vi "setControlTargetPosition.vi"(8 "error":errorcluster, 9 "target":dbl format="%#_13g", 10 "axis":i32, 11 "connection ID":refnum<k5>) -> (0 "error out":errorcluster, 2 "axis_out":i32, 3 "connection ID out":refnum<k5>)   [LabVIEW 2016, in "amc_api.lvlib"]
doc: "This function sets the target position for the movement on the selected axis."
uses:
  amc_api.lvlib
panel:
  out "jsonRespIn":string
  out "JSON-response":string="{\"jsonrpc\":\"2.0\",\"method\":\"\",\"params\":[5,1.245,true,\"name\"],\"id\":\"1\"}"
  out "JSON request":string
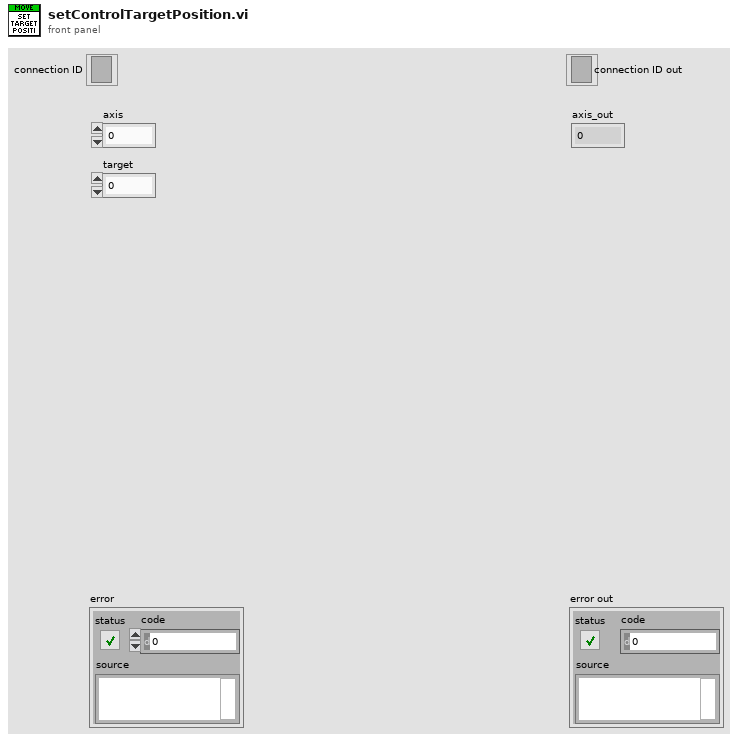
[diagram p1: front panel]
types:
  T1 = cluster{"jsonrpc":string, "method":string, "params":string[], "id":string, "api":i32, "pid":string}
  T2 = enum16{"Standard", "Buffered", "CRLF", "Immediate"}
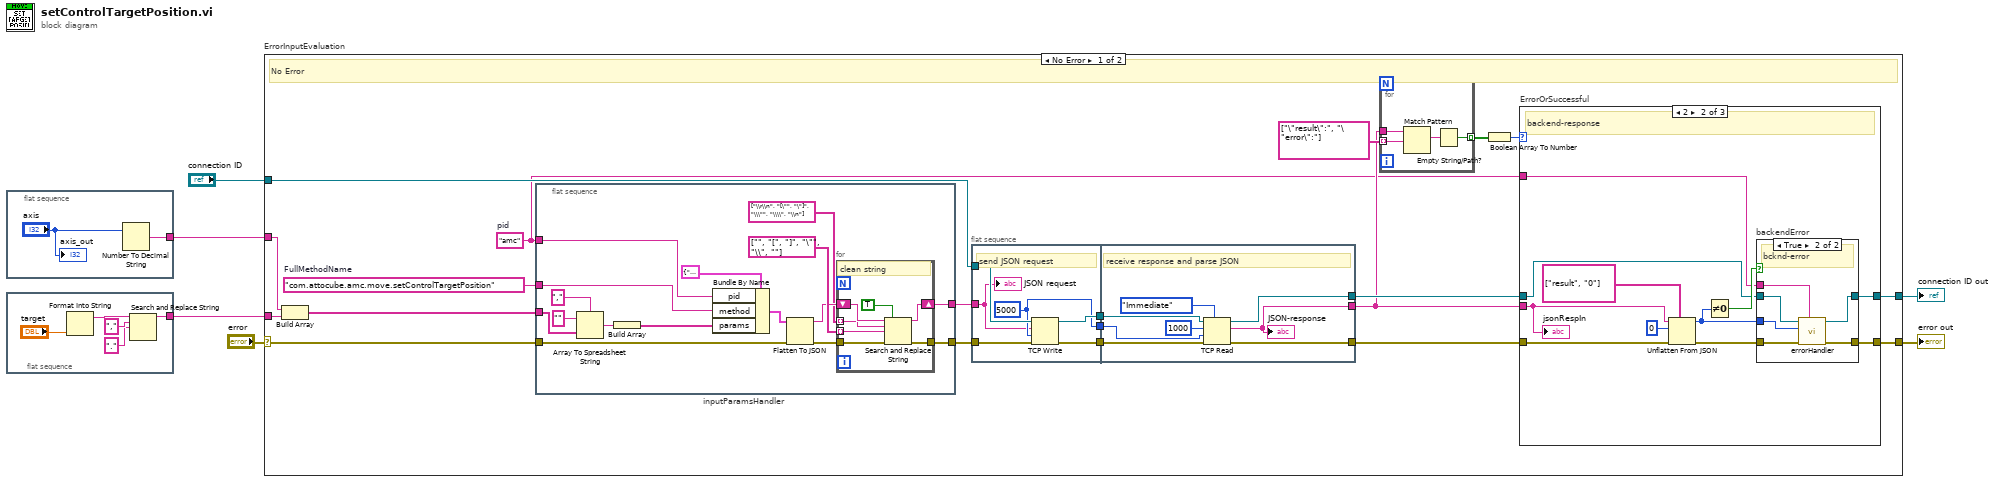
[diagram p0: block diagram]
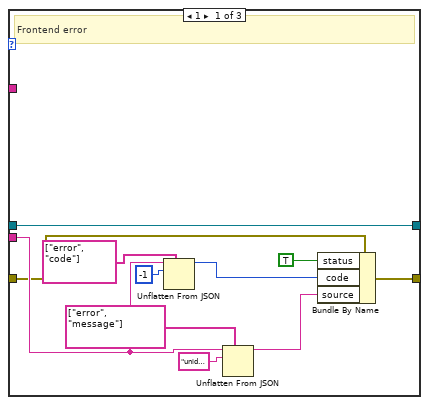
[diagram p2: hidden frame]
diagram:
  n1 = flat-sequence "in_axis" {
    tunnel: [w8] -> w2
    frame #0 {
      n2 = Number To Decimal String(number="axis") -> (decimal integer string=w8:string)  [unwired: 1 in]
      "axis_out" <- "axis"
    }
  }
  n3 = flat-sequence "in_double" {
    tunnel: [w9] -> w1
    frame #0 {
      n4 = Format Into String("target") -> (resulting string=w12:string)  [unwired: 3 in, 1 out]
      n5 = Search and Replace String(input string=w12, search string=",", replace string="." ("search string")) -> (result string=w9:string)  [unwired: 5 in, 3 out]
    }
  }
  n6 = case "ErrorInputEvaluation" shown="No Error" "error" {
    selector: "error" -> [w20 w107]
    tunnel: "connection ID" -> [w30 w108]
    tunnel: [w22 w107] -> w5
    tunnel: [w23 w108] -> w4
    tunnel: w2 -> [w15 _]
    tunnel: w1 -> [w14 _]
    frame No Error {
      w16 = "amc"  # pid
      w21 = "com.attocube.amc.move.setControlTargetPosition"  # FullMethodName
      # "No Error"
      n7 = Build Array ("ParametersArrayString")(w15, w14) -> (w19:string[])
      n8 = flat-sequence "inputParamsHandler" {
        tunnel: [w39] -> w18
        tunnel: w19 -> [w45]
        tunnel: w20 -> [w44]
        tunnel: [w41] -> w17
        tunnel: w21 -> [w35]
        tunnel: w16 -> [w34]
        frame #0 {
          n9 = Array To Spreadsheet String(delimiter (Tab)=",", array=w45, 3:"" ("format string")) -> (spreadsheet string=w47:string)
          n10 = Build Array "Build Array"(w47) -> (w36:string[])
          n11 = Bundle By Name(cluster=T1 {"jsonrpc"="2.0", "method"="com.attocube.amc.res.setRESReadOutFreq", "params"=[], "id"="1", "api"=2, "pid"=""}, "pid"=w34, "method"=w35, "params"=w36) -> (w46:T1)
          n12 = Flatten To JSON(anything=w46, error in (no error)=w44) -> (JSON string=w40:string, 11:w42:errorcluster)  [unwired: 1 in]
          n13 = for {
            tunnel: string[] ["\\r\\n", "[\"", "\"]", "\\\"", "\\\\", "\\n"] ("search string") -> [w53] mode=indexing
            tunnel: string[] ["", "[", "]", "\"", "\\", ""] ("replace string (\"\")") -> [w52] mode=indexing
            shift-right: [w55] -> w39
            shift-left: w40 -> [w54]
            tunnel: w42 -> [w51]
            tunnel: [w50] -> w41
            # "clean string"
            n14 = Search and Replace String(replace all?=TRUE ("replace all? (F)"), input string=w54, search string=w53, replace string=w52, error in=w51) -> (result string=w55:string, error out=w50:errorcluster)  [unwired: 3 in, 2 out]
          }
        }
      }
      n15 = flat-sequence {
        tunnel: w30 -> [w98]
        tunnel: [w96] -> w33
        tunnel: [w97] -> w32
        tunnel: w17 -> [w93]
        tunnel: [w95] -> w31
        tunnel: w18 -> [w94]
        tunnel: [w102] -> w26
        tunnel: w33 -> [w104]
        tunnel: w32 -> [w103]
        tunnel: [w100] -> w25
        tunnel: w31 -> [w101]
        tunnel: [w99] -> w24
        frame #0 {
          w95 = 5000 ("timeout ms (25000)")
          # "send JSON request"
          n16 = TCP Write(connection ID=w98, data in=w94, error in (no error)=w93, 9:w95) -> (connection ID out=w96:refnum<k5>, error out=w97:errorcluster)  [unwired: 1 out]
          "JSON request" <- w94
        }
        frame #1 {
          # "receive response and parse JSON"
          n17 = TCP Read(connection ID=w104, bytes to read=1000, error in (no error)=w103, 7:T2."Immediate" ("mode (standard)"), 9:w101) -> (connection ID out=w102:refnum<k5>, data out=w99:string, error out=w100:errorcluster)
          "JSON-response" <- w99
        }
      }
      n18 = for {
        tunnel: string[] ["\"result\":", "\"error\":"] ("path") -> [w59] mode=indexing
        tunnel: [w57] -> w28 mode=indexing
        tunnel: w24 -> [w60]
        n19 = Match Pattern(string=w60, regular expression=w59) -> (match substring=w58:string)  [unwired: 1 in, 3 out]
        n20 = Empty String/Path?(string/path=w58) -> (empty?=w57:bool)
      }
      n21 = Boolean Array To Number(Boolean array=w28) -> (number=w27:u32)
      n22 = case "ErrorOrSuccessful" shown="2" w27 {
        tunnel: w24 -> [w63 w73 _]
        tunnel: w26 -> [w61 w76 w92]
        tunnel: [w61 w75 w92] -> w23
        tunnel: [w64 w74 w91] -> w22
        tunnel: w25 -> [w62 w77 w91]
        tunnel: w16 -> [_ w72 _]
        frame 1 {
          # "Frontend error"
          n23 = Unflatten From JSON(path=string[] ["error", "code"], JSON string=w63, type and defaults=-1) -> (value=w70:i32)  [unwired: 4 in, 1 out]
          n24 = Unflatten From JSON(path=string[] ["error", "message"], JSON string=w63, type and defaults="unidentified error") -> (value=w71:string)  [unwired: 4 in, 1 out]
          n25 = Bundle By Name(cluster=w62, "status"=TRUE, "code"=w70, "source"=w71) -> (w64:errorcluster)
        }
        frame 2 {
          # "backend-response"
          n26 = Unflatten From JSON(path=string[] ["result", "0"], JSON string=w73, type and defaults=0, error in (no error)=w77) -> (value=w82:i32, error out=w80:errorcluster)  [unwired: 3 in]
          n27 = Not Equal To 0?(x=w82) -> (x != 0?=w81:bool)
          n28 = case "backendError" shown="True" w81 {
            tunnel: w82 -> [_ w90]
            tunnel: w80 -> [w84 w89]
            tunnel: [w83 w88] -> w75
            tunnel: [w84 w87] -> w74
            tunnel: w76 -> [w83 w86]
            tunnel: w72 -> [_ w85]
            frame False {
              # "successful"
            }
            frame True {
              # "bcknd-error"
              n29 = call "errorHandler.vi"("pid"=w85, "error in"=w89, "errNbr"=w90, "connection ID"=w86) -> ("error out 2"=w87:errorcluster, "connection ID out"=w88:refnum<k5>)  [unwired: 6 in]
            }
          }
          "jsonRespIn" <- w73
        }
        frame Default {
          # "NoResponse"
        }
      }
    }
    frame Error {
      # "Error"
    }
  }
  "error out" <- w5
  "connection ID out" <- w4
